vi "Client Subscription Integration Test.vi"() -> (0 "error out":errorcluster)   [LabVIEW 2024]
uses:
  src/NATS Client/NATS Client.lvclass/NATS Client.ctl
  <vilib>/NATS/NATS Core/VIs/NATS CLOSE.vi
  src/NATS Client/get async stop notifier.vi
  src/NATS Client/Get Connection DVR.vi
  src/NATS Client/get subscriptions queue.vi
  src/NATS Client/Get subscription map.vi
  src/NATS Client/Get error queue.vi
  <vilib>/addons/_JKI Toolkits/Caraya/classes/Assert/Assert True.vi
  <vilib>/addons/_JKI Toolkits/Caraya/classes/Assert/Assert Equal Value and Type_Variant.vi
  <vilib>/addons/_JKI Toolkits/Caraya/classes/Assert/Assert False.vi
  <vilib>/addons/_JKI Toolkits/Caraya/classes/Assert/Assert Error.vi
  <vilib>/addons/_JKI Toolkits/Caraya/classes/Assert/Assert Equal Value_Variant.vi
  src/NATS Subscription/NATS Subscription.lvclass
  <vilib>/addons/_JKI Toolkits/Caraya/classes/Test/Test.lvclass
  src/NATS Client/NATS Client.lvclass
  <vilib>/addons/_JKI Toolkits/Caraya/classes/Assert/Assert.lvclass
  src/NATS Infrastructure/NATS Infrastructure.lvlib
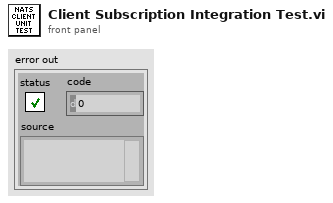
[diagram p1: front panel]
types:
  T1 = typedef "NATS Core.lvlib/nats message.ctl" = cluster{"subject":string, "payload":string, "sub id":string, "reply-to":string, "headers":string, "type":T2, "received":timestamp}
  T2 = typedef "NATS Core.lvlib/msg type.ctl" = enum16{"Undefined", "MSG", "HMSG", "+OK", "PING", "PONG", "-ERR", "INFO"}
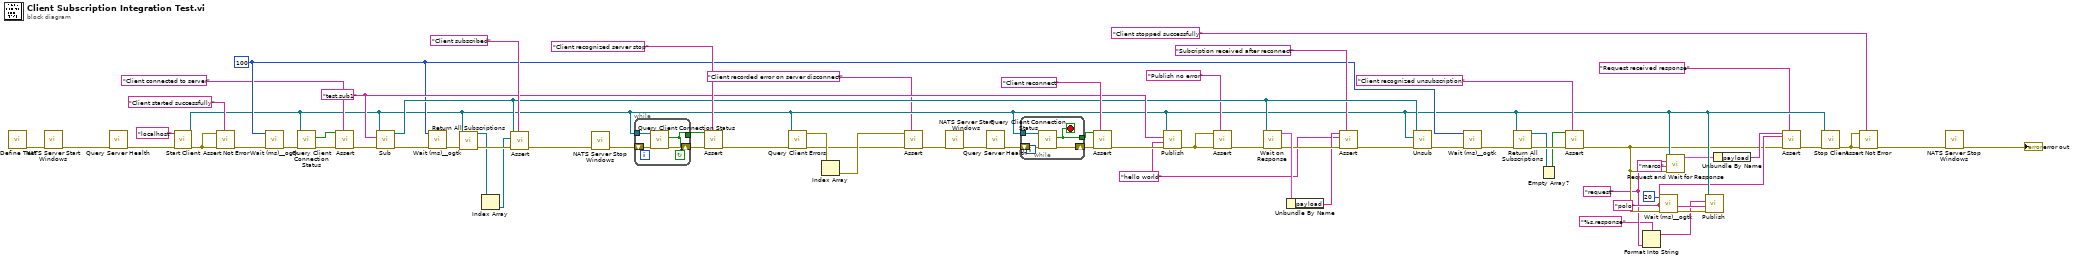
[diagram p0: block diagram]
diagram:
  w3 = "request" ("subject")
  w10 = "polo" ("payload")
  w34 = "hello world" ("payload")
  w22 = u32 100 ("milliseconds to wait")
  w40 = "test.sub1" ("subject")
  n1 = call <vilib>:"Define Test.vi"() -> ("error out"=w64:errorcluster)  [unwired: 10 in, 1 out]
  n2 = call "NATS Server Start Windows.vi"("error in"=w64) -> ("error out"=w63:errorcluster)  [unwired: 10 in]
  n3 = call "Query Server Health.vi"("error in"=w63) -> ("error out"=w61:errorcluster)  [unwired: 9 in, 1 out]
  n4 = call "Start Client.vi"("error in"=w61, "address"="localhost") -> ("error out"=w69:errorcluster, "NATS Client out"=w14:refnum<class "NATS Client.lvclass">)  [unwired: 8 in]
  n5 = call <vilib>:"Assert Not Error.vi"("Label"="Client started successfully", "error in (no error)"=w69, "Not Error?"=w69) -> ("error out"=w60:errorcluster)  [unwired: 7 in, 1 out]
  n6 = call <userlib>:"Wait (ms)__ogtk.vi"("error in (no error)"=w60, "milliseconds to wait"=w22) -> ("error out"=w56:errorcluster)  [unwired: 8 in, 1 out]
  n7 = call "Query Client Connection Status.vi"("error in"=w56, "NATS Client in"=w14) -> ("error out"=w58:errorcluster, "Connected"=w59:bool)  [unwired: 8 in]
  n8 = call-poly <vilib>:"Assert.vi"("Label"="Client connected to server", "error in (no error)"=w58, "True?"=w59) -> ("error out"=w55:errorcluster)  [unwired: 7 in, 1 out]
  n9 = call "Sub.vi"("error in"=w55, "subject"=w40, "NATS Client"=w14) -> ("error out"=w52:errorcluster, "NATS Subscription"=w33:refnum<class "NATS Subscription.lvclass">)  [unwired: 7 in]
  n10 = call <userlib>:"Wait (ms)__ogtk.vi"("error in (no error)"=w52, "milliseconds to wait"=w22) -> ("error out"=w46:errorcluster)  [unwired: 8 in, 1 out]
  n11 = call "Return All Subscriptions.vi"("error in"=w46, "NATS Client"=w14) -> ("error out"=w57:errorcluster, "Subscriptions"=w54:refnum<class "NATS Subscription.lvclass">[])  [unwired: 8 in]
  n12 = Index Array(array=w54) -> (element=w53:refnum<class "NATS Subscription.lvclass">)  [unwired: 1 in]
  n13 = call-poly <vilib>:"Assert.vi"("Label"="Client subscribed", "error in (no error)"=w57, "Actual"=w53, "Expected"=w33) -> ("error out"=w51:errorcluster)  [unwired: 6 in, 1 out]
  n14 = call "NATS Server Stop Windows.vi"("error in"=w51) -> ("error out"=w21:errorcluster)  [unwired: 10 in]
  n15 = while {
    tunnel: [w72] -> w44
    shift-right: [w74] -> w50
    shift-left: w21 -> [w73]
    tunnel: w14 -> [w71]
    stop <- w72 continue-if-true
    n16 = call "Query Client Connection Status.vi"("error in"=w73, "NATS Client in"=w71) -> ("error out"=w74:errorcluster, "Connected"=w72:bool)  [unwired: 8 in]
  }
  n17 = call-poly <vilib>:"Assert.vi"("Label"="Client recognized server stop", "error in (no error)"=w50, "False?"=w44) -> ("error out"=w45:errorcluster)  [unwired: 7 in, 1 out]
  n18 = call "Query Client Errors.vi"("error in"=w45, "NATS Client"=w14) -> ("error out"=w15:errorcluster, "errors"=w17:errorcluster[])  [unwired: 8 in]
  n19 = Index Array(array=w17) -> (element=w16:errorcluster)  [unwired: 1 in]
  n20 = call-poly <vilib>:"Assert.vi"("Label"="Client recorded error on server disconnect", "error in (no error)"=w15, "Error?"=w16) -> ("error out"=w18:errorcluster)  [unwired: 7 in, 1 out]
  n21 = call "NATS Server Start Windows.vi"("error in"=w18) -> ("error out"=w49:errorcluster)  [unwired: 10 in]
  n22 = call "Query Server Health.vi"("error in"=w49) -> ("error out"=w20:errorcluster)  [unwired: 9 in, 1 out]
  n23 = while {
    tunnel: [w75] -> w47
    shift-right: [w78] -> w48
    shift-left: w20 -> [w77]
    tunnel: w14 -> [w76]
    stop <- w75 stop-if-true
    n24 = call "Query Client Connection Status.vi"("error in"=w77, "NATS Client in"=w76) -> ("error out"=w78:errorcluster, "Connected"=w75:bool)  [unwired: 8 in]
  }
  n25 = call-poly <vilib>:"Assert.vi"("Label"="Client reconnect", "error in (no error)"=w48, "True?"=w47) -> ("error out"=w39:errorcluster)  [unwired: 7 in, 1 out]
  n26 = call "Publish.vi"("error in"=w39, "payload"=w34, "subject"=w40, "NATS Client.lvlib:NATS Client.lvclass"=w14) -> ("error out"=w25:errorcluster)  [unwired: 7 in]
  n27 = call-poly <vilib>:"Assert.vi"("Label"="Publish no error", "error in (no error)"=w25, "Not Error?"=w25) -> ("error out"=w26:errorcluster)  [unwired: 7 in, 1 out]
  n28 = call "Wait on Response.vi"("error in"=w26, "NATS Subscriber in"=w33) -> ("error out"=w36:errorcluster, "nats message"=w38:T1)  [unwired: 7 in, 1 out]
  n29 = Unbundle By Name(w38) -> ("payload"=w35:string)
  n30 = call-poly <vilib>:"Assert.vi"("Label"="Subcription received after reconnect", "error in (no error)"=w36, "Actual"=w34, "Expected"=w35) -> ("error out"=w37:errorcluster)  [unwired: 6 in, 1 out]
  n31 = call "Unsub.vi"("error in"=w37, "NATS Client"=w14, "NATS Subscription"=w33) -> ("error out"=w31:errorcluster)  [unwired: 7 in, 1 out]
  n32 = call <userlib>:"Wait (ms)__ogtk.vi"("error in (no error)"=w31, "milliseconds to wait"=w22) -> ("error out"=w27:errorcluster)  [unwired: 8 in, 1 out]
  n33 = call "Return All Subscriptions.vi"("error in"=w27, "NATS Client"=w14) -> ("error out"=w32:errorcluster, "Subscriptions"=w30:refnum<class "NATS Subscription.lvclass">[])  [unwired: 8 in]
  n34 = Empty Array?(array=w30) -> (empty?=w29:bool)
  n35 = call-poly <vilib>:"Assert.vi"("Label"="Client recognized unsubscription", "error in (no error)"=w32, "True?"=w29) -> ("error out"=w8:errorcluster)  [unwired: 7 in, 1 out]
  n36 = Format Into String(format string="%s.response", w3) -> (resulting string=w1:string)  [unwired: 2 in, 1 out]
  n37 = call <userlib>:"Wait (ms)__ogtk.vi"("error in (no error)"=w8, "milliseconds to wait"=u32 20) -> ("error out"=w7:errorcluster)  [unwired: 8 in, 1 out]
  n38 = call "Request and Wait for Response.vi"("error in"=w8, "payload"="marco", "subject"=w3, "NATS Client in"=w14) -> ("nats message"=w13:T1)  [unwired: 5 in, 2 out]
  n39 = call "Publish.vi"("error in"=w7, "payload"=w10, "subject"=w1, "NATS Client.lvlib:NATS Client.lvclass"=w14) -> ()  [unwired: 7 in, 1 out]
  n40 = Unbundle By Name(w13) -> ("payload"=w11:string)
  n41 = call-poly <vilib>:"Assert.vi"("Label"="Request received response", "error in (no error)"=w8, "Actual"=w10, "Expected"=w11) -> ("error out"=w12:errorcluster)  [unwired: 6 in, 1 out]
  n42 = call "Stop Client.vi"("error in"=w12, "NATS Client"=w14) -> ("error out"=w67:errorcluster)  [unwired: 9 in]
  n43 = call <vilib>:"Assert Not Error.vi"("Label"="Client stopped successfully", "error in (no error)"=w67, "Not Error?"=w67) -> ("error out"=w65:errorcluster)  [unwired: 7 in, 1 out]
  n44 = call "NATS Server Stop Windows.vi"("error in"=w65) -> ("error out"=→"error out":errorcluster)  [unwired: 10 in]
